vi "Temperature Monitor PC.vi"() -> ()   [LabVIEW 2010]
panel:
  out "Temperature History (C)":sgl(graph)
  in  "Stop Windows GUI":bool
  out "Temperature Alarm":bool
  in  "Temperature\nAlarm Level (C)":sgl(slide)=30.0 caption="Temperature Alarm Level (C)" scale=20.0..50.0
  in  "Save File Path":path=path "C:/Exercises/FPGA/RT Host and PC Integration/Temp Data.lvm" caption="File Name"
  in  "Sample Interval (ms)":u32(knob)=500 scale=10.0..1000.0
  in  "Stop RT":bool
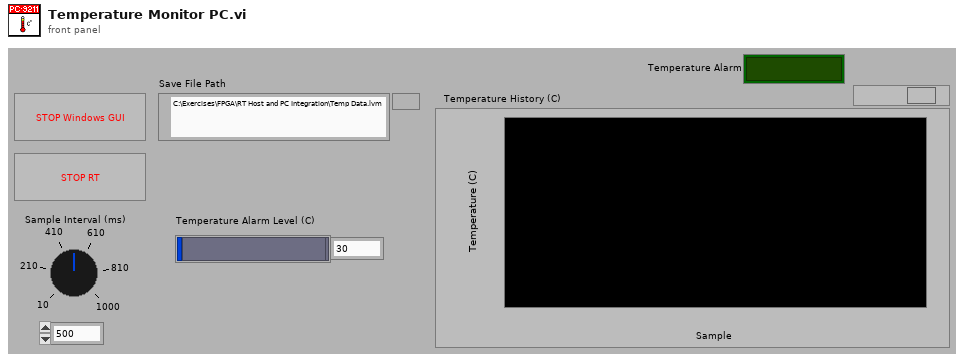
[diagram p1: front panel]
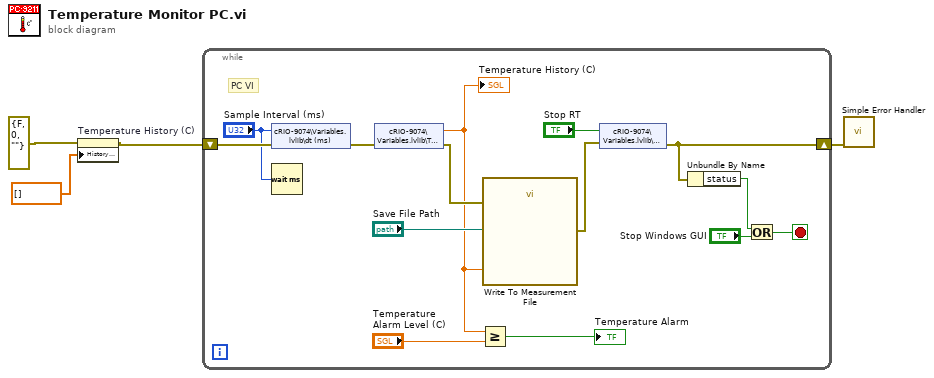
[diagram p0: block diagram]
diagram:
  n1 = property on="Temperature History (C)" class="WFChart (strict)"(error in=errorcluster {"status"=FALSE, "code"=0, "source"=""} ("error in (no error)"), "History Data"=sgl[] []) -> (error out=w1:errorcluster)  [unwired: 1 in, 1 out]
  n2 = while {
    shift-right: [w11] -> w4
    shift-left: w1 -> [w18]
    stop <- w12 stop-if-true
    # "PC VI"
    n3 = shared-variable "cRIO-9074\\Variables.lvlib\\dt (ms)"("Sample Interval (ms)", error in=w18) -> (error out=w6:errorcluster)
    n4 = Wait (ms)(milliseconds to wait="Sample Interval (ms)") -> ()  [unwired: 1 out]
    n5 = shared-variable "cRIO-9074\\Variables.lvlib\\T (C)"(error in=w6) -> (w5:sgl, error out=w9:errorcluster)
    "Temperature History (C)" <- w5
    n6 = Greater Or Equal?(x=w5, y="Temperature\nAlarm Level (C)") -> (x >= y?=→"Temperature Alarm":bool)
    n7 = call "Write To Measurement File"("Signals"=w5, "error in (no error)"=w9, "Filename"="Save File Path") -> ("error out"=w8:errorcluster)  [unwired: 14 in, 2 out]
    n8 = shared-variable "cRIO-9074\\Variables.lvlib\\Stop"("Stop RT", error in=w8) -> (error out=w11:errorcluster)
    n9 = Unbundle By Name(w11) -> ("status"=w10:bool)
    n10 = Or(x=w10, y="Stop Windows GUI") -> (x .or. y?=w12:bool)
  }
  n11 = call <vilib>:"Simple Error Handler.vi"("error in (no error)"=w4) -> ()  [unwired: 1 in, 8 out]
